vi "CalcMotorTorque.vi"(9 "Motor Characteristics":T1, 10 "Motor Current":dbl, 11 "Motor Voltage":dbl) -> (3 "Motor Torque":dbl)   [LabVIEW 2014]
panel:
  in  "Reference Voltage (12)":dbl=12.0
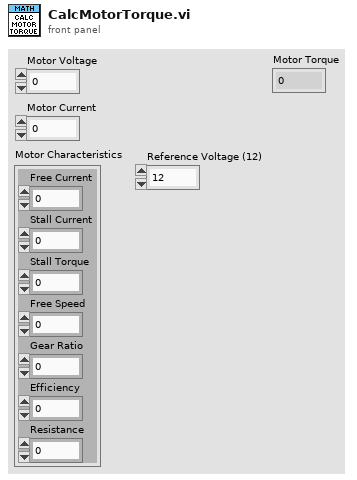
[diagram p1: front panel]
types:
  T1 = cluster{"Free Current":dbl, "Stall Current":dbl, "Stall Torque":dbl, "Free Speed":dbl, "Gear Ratio":dbl, "Efficiency":dbl, "Resistance":dbl}
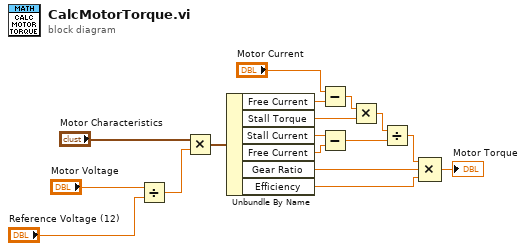
[diagram p0: block diagram]
diagram:
  n1 = Divide(x="Motor Voltage", y="Reference Voltage (12)") -> (x/y=w16:dbl)
  n2 = Multiply(x="Motor Characteristics", y=w16) -> (x*y=w15:T1)
  n3 = Unbundle By Name(w15) -> ("Free Current"=w14:dbl, "Stall Torque"=w12:dbl, "Stall Current"=w11:dbl, "Free Current"=w10:dbl, "Gear Ratio"=w6:dbl, "Efficiency"=w5:dbl)
  n4 = Subtract(x="Motor Current", y=w14) -> (x-y=w13:dbl)
  n5 = Subtract(x=w11, y=w10) -> (x-y=w8:dbl)
  n6 = Multiply(x=w13, y=w12) -> (x*y=w9:dbl)
  n7 = Divide(x=w9, y=w8) -> (x/y=w7:dbl)
  n8 = Compound Arithmetic op=MULTIPLY(w7, w6, w5) -> (→"Motor Torque":dbl)
